vi "Traffic Monitoring Hub.vi"() -> ()   [LabVIEW 2017]
uses:
  <vilib>/LabVIEW Open Source Project/MQTT Broker/Client/Client.lvclass
  C:/Program Files (x86)/National Instruments/LabVIEW 2017/vi.lib/LabVIEW Open Source Project/MQTT Broker/MQTT_Base/MQTT_Base.lvclass
  <vilib>/LabVIEW Open Source Project/MQTT Broker/Control Packets/PUBLISH/PUBLISH.lvclass
  C:/Program Files (x86)/National Instruments/LabVIEW 2017/vi.lib/LabVIEW Open Source Project/MQTT Broker/Control Packets/ControlPacket/ControlPacket.lvclass
  <vilib>/LabVIEW Open Source Project/MQTT Broker/Client/Client.lvclass/Client.ctl
  <vilib>/LabVIEW Open Source Project/MQTT Broker/Control Packets/ControlPacket/ControlPacket.lvclass/ControlPacket.ctl
  0d705227-134d-4031-8d1e-e35da49b8ba8.vi
  89a43b97-b5cf-4dc9-9f30-016ac9be9430.vi
  45bbbbd6-bbd6-4c9d-8aa1-54a553140d59.vi
  b830538a-2e83-4cc7-9605-dce1a29f0d38.vi
  <vilib>/LabVIEW Open Source Project/MQTT Broker/MQTT_Base/Decode Publish Package.vi
  <vilib>/LabVIEW Open Source Project/MQTT Broker/MQTT_Base/MQTT_Base.lvclass
  <vilib>/LabVIEW Open Source Project/MQTT Broker/Control Packets/ControlPacket/ControlPacket.lvclass
panel:
  in  "Destroy Sim Cars":bool
  in  "Generate Sim Cars":bool
  in  "# Cars":i32=10
  out "Will Message":string
  out "last update":timestamp
  out "Payload":variant
  in  "State History":i32(listbox)
  out "Topic":string
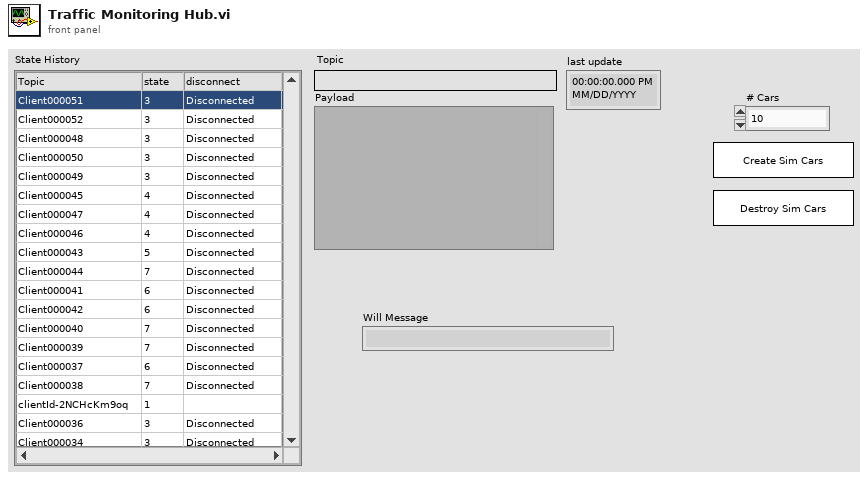
[diagram p1: front panel]
types:
  T1 = enum32{"Invalid", "Standard", "Closed", "Hidden", "Minimized", "Maximized"}
  T2 = enum32{"invalid app kind", "Development System", "Run Time System", "Student Edition", "Embedded LabVIEW", "Evaluation", "Custom"}
  T3 = cluster{"Core":cluster{"Current VI Reference":refnum<vi>, "Close Panel on Exit?":bool}, "server address":string, "project namespace":string, "Client Name":string, "Client":refnum<class "Client.lvclass">, "Close on MQTT Disconnection?":bool, "Subscription":string, "AppMessage":refnum<class "PUBLISH.lvclass">, "stop signal":refnum<user-event>}
  T4 = cluster{"Current VI Reference":refnum<vi>, "Close Panel on Exit?":bool}
  T5 = typedef "MQTT Server.lvlib/Client.lvclass/Public Events -- cluster.ctl" = cluster{"Connection Status":refnum<user-event>, "Connected":refnum<user-event>, "Application Message":refnum<user-event>}
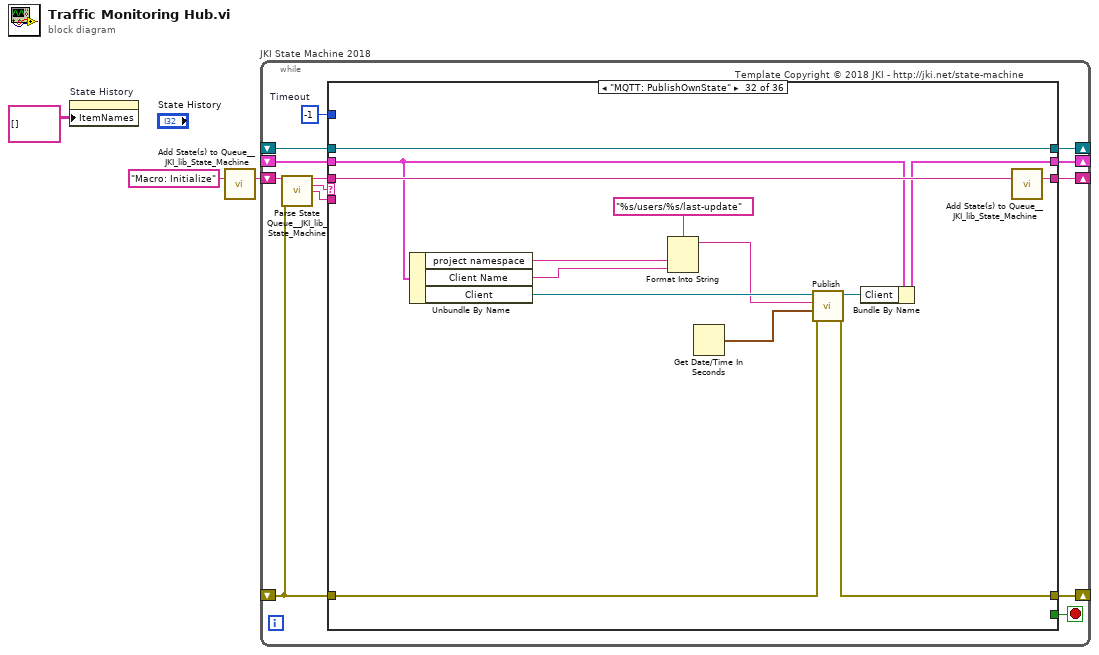
[diagram p0: block diagram]
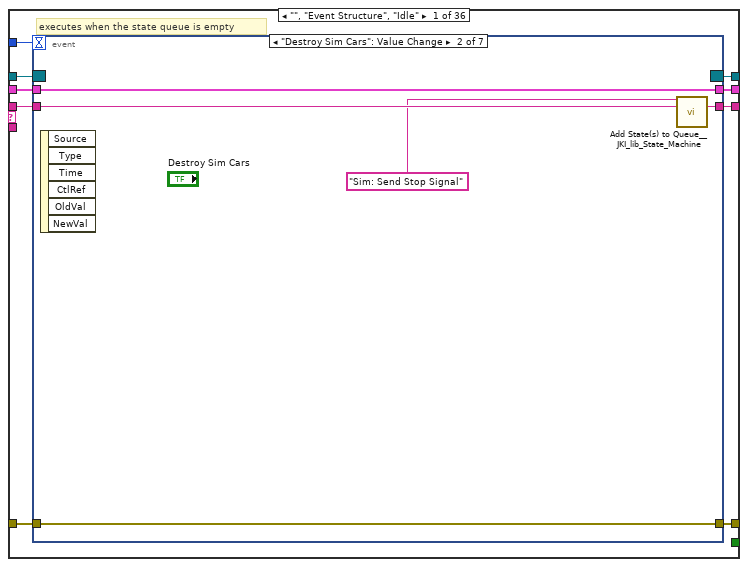
[diagram p2: hidden frame]
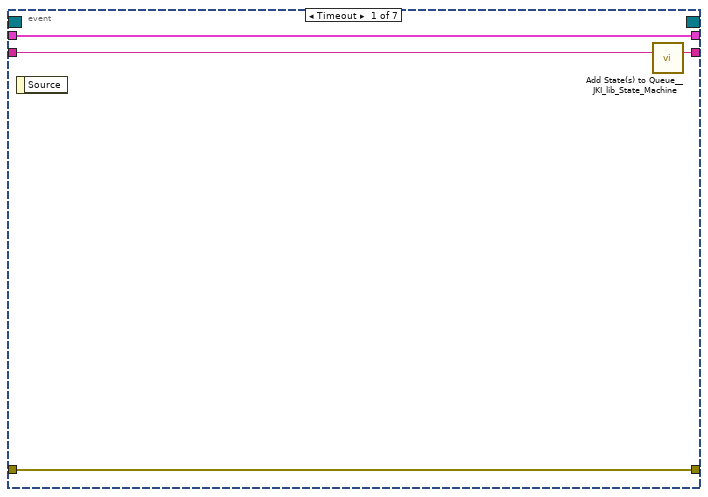
[diagram p3: hidden frame]
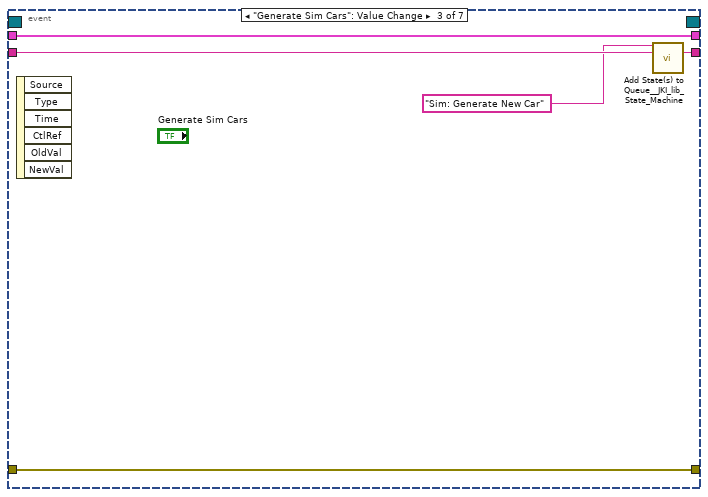
[diagram p4: hidden frame]
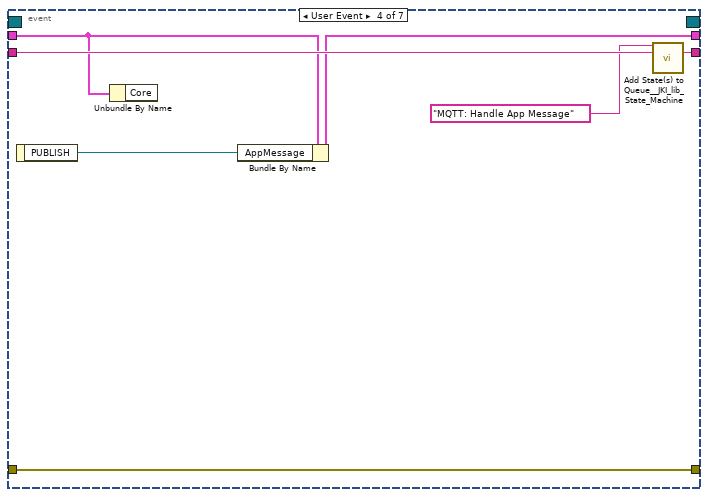
[diagram p5: hidden frame]
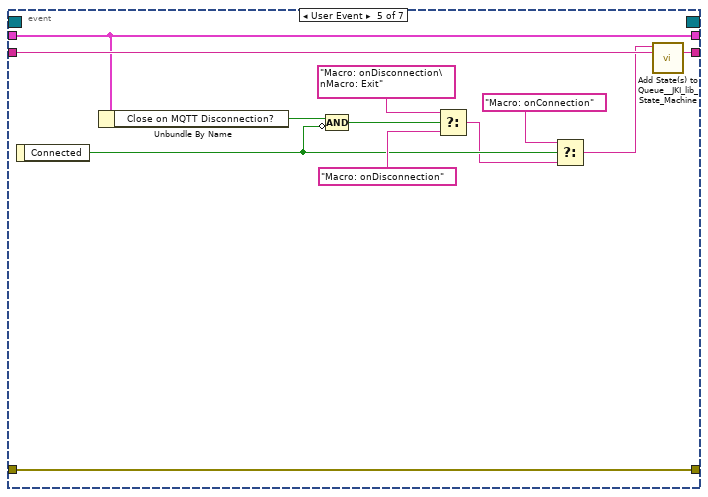
[diagram p6: hidden frame]
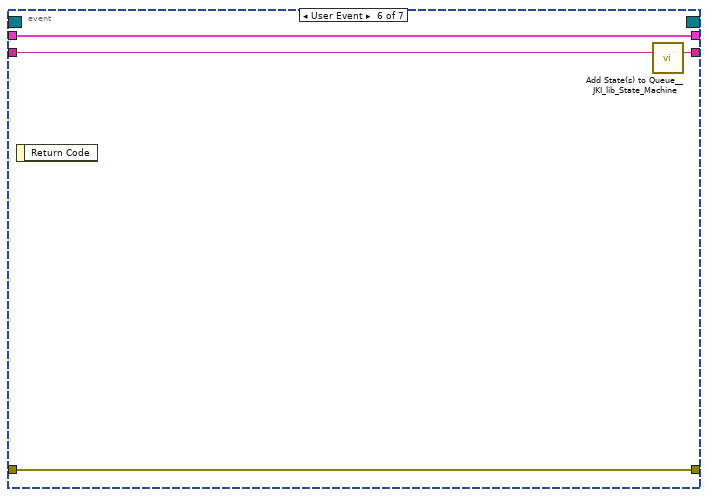
[diagram p7: hidden frame]
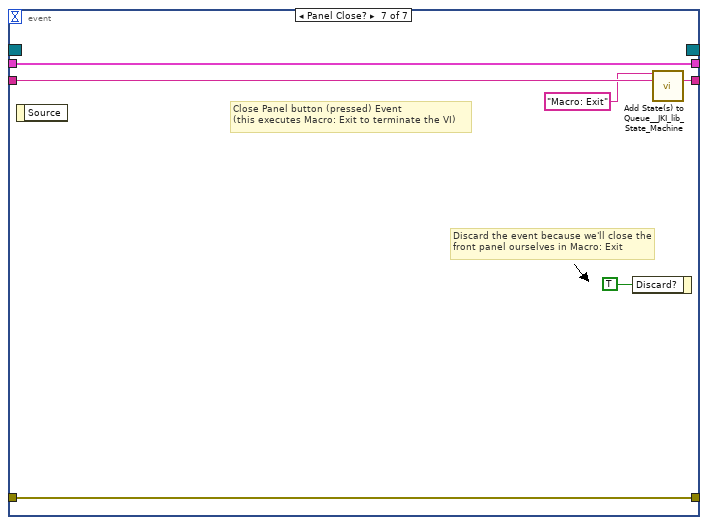
[diagram p8: hidden frame]
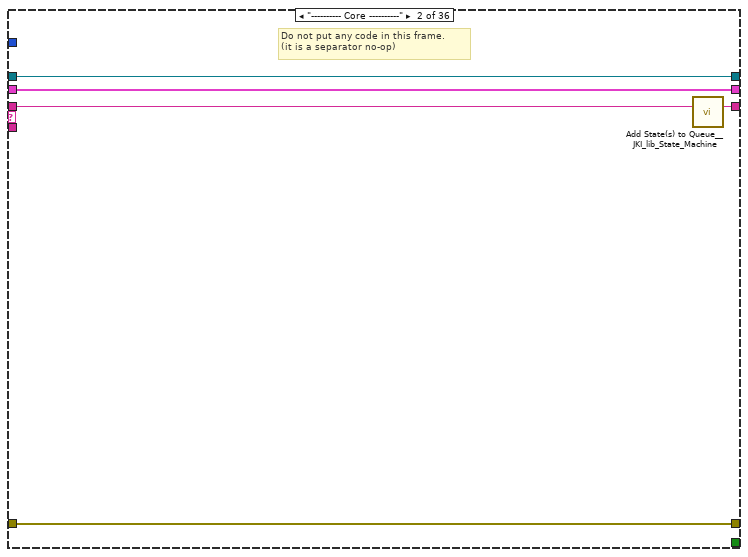
[diagram p9: hidden frame]
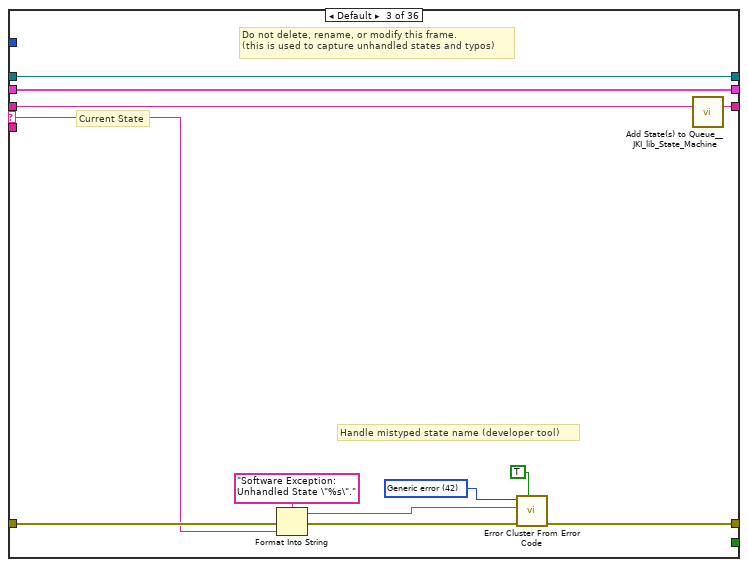
[diagram p10: hidden frame]
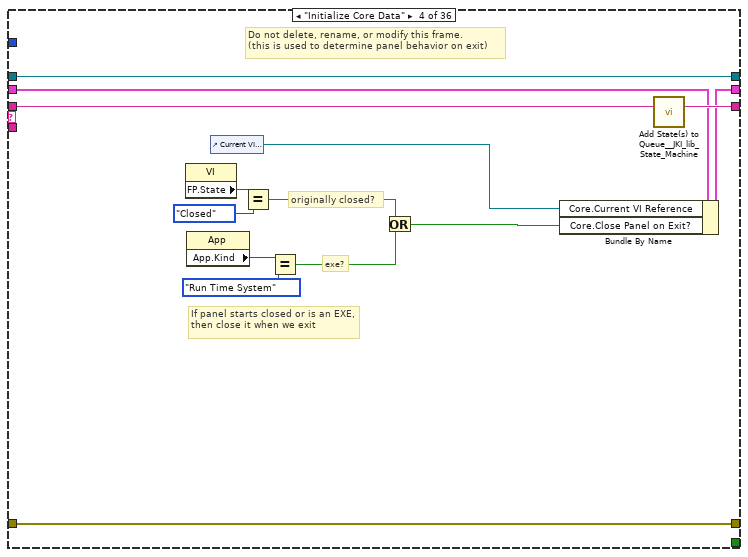
[diagram p11: hidden frame]
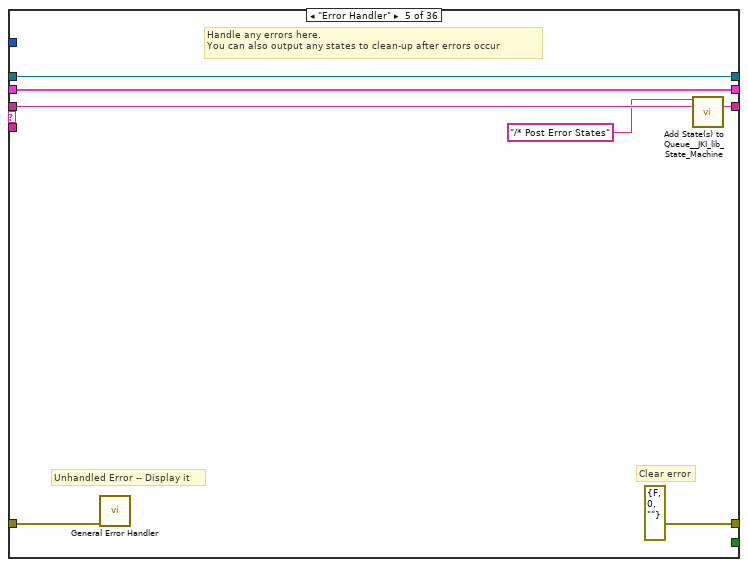
[diagram p12: hidden frame]
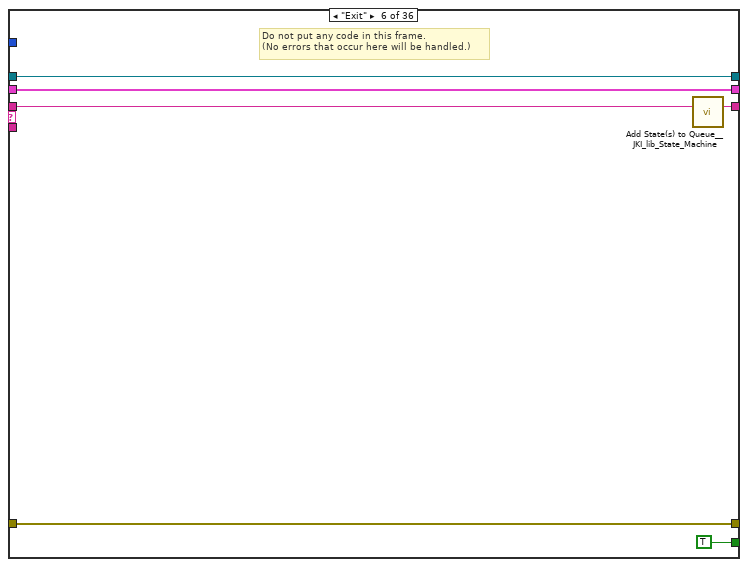
[diagram p13: hidden frame]
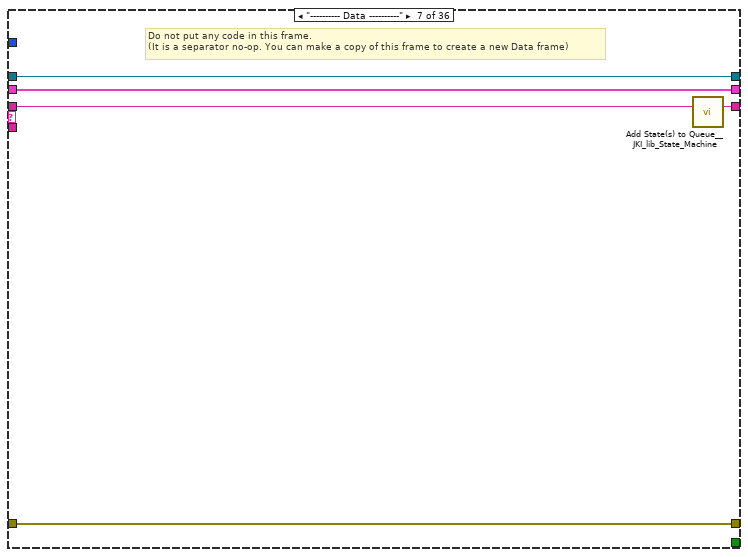
[diagram p14: hidden frame]
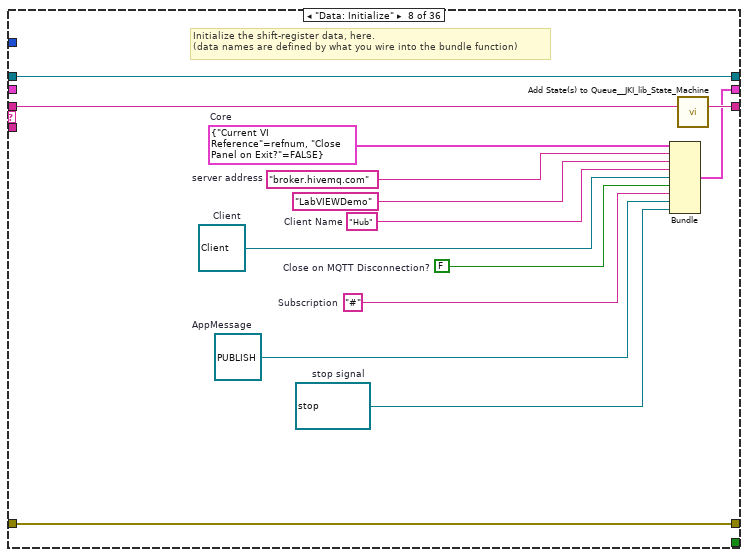
[diagram p15: hidden frame]
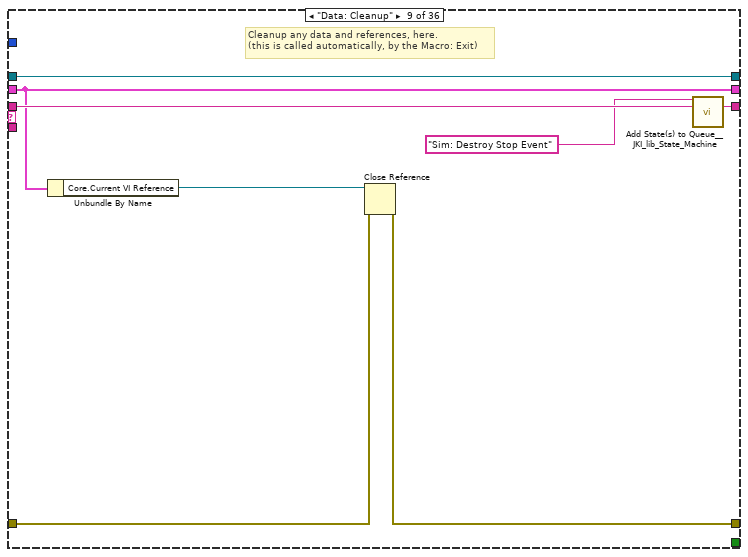
[diagram p16: hidden frame]
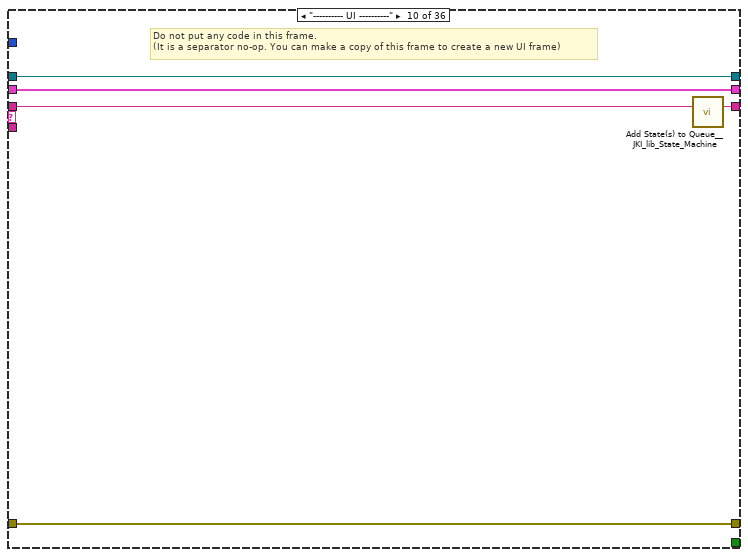
[diagram p17: hidden frame]
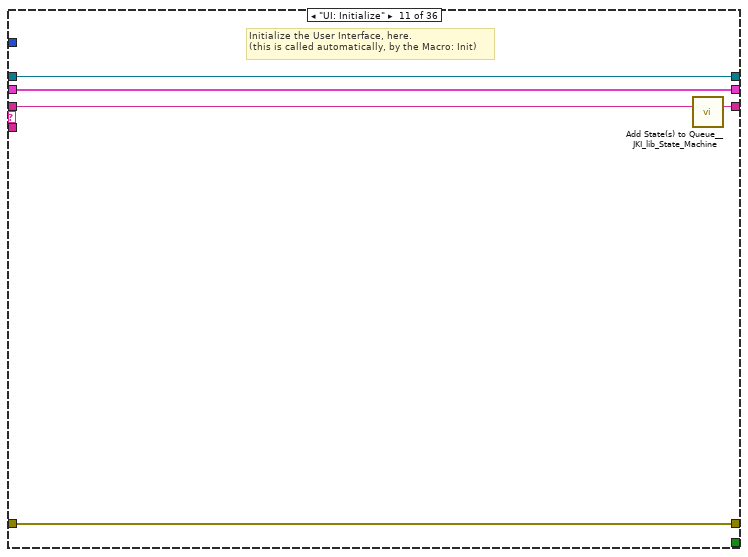
[diagram p18: hidden frame]
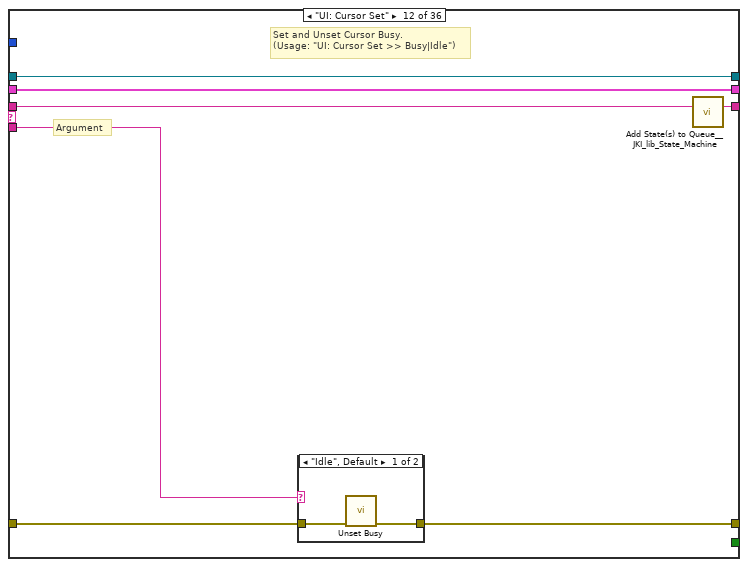
[diagram p19: hidden frame]
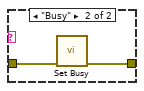
[diagram p20: hidden frame]
diagram:
  n1 = property on="State History" class="MCListbox (strict)"("ItemNames"=string[][] [] ("Item Names")) -> ()  [unwired: 2 in, 2 out]
  n2 = call <vilib>:"Add State(s) to Queue__JKI_lib_State_Machine.vi"("State(s) in (\"\")"="Macro: Initialize") -> ("States Out"=w2:string)  [unwired: 14 in]
  n3 = while "JKI State Machine 2018" {
    shift-right: [w9] -> _
    shift-left: _ -> [w8]
    shift-right: [w12] -> _
    shift-left: _ -> [w6]
    shift-right: [w11] -> _
    shift-left: w2 -> [w13]
    shift-right: [w4] -> _
    shift-left: _ -> [w5]
    stop <- w10 stop-if-true
    w7 = -1  # Timeout
    # "Template Copyright © 2018 JKI - http://jki.net/state-machine"
    n4 = call <vilib>:"Parse State Queue__JKI_lib_State_Machine.vi"("State Queue"=w13, "Error In (no error)"=w6) -> ("Remaining States"=w15:string, "Current State"=w16:string, "Arguments"=w14:string)  [unwired: 11 in]
    n5 = case shown="\"MQTT: PublishOwnState\"" w16 {
      selector: w16 -> [_ _ w75 _ _ _ _ _ _ _ _ _ _ _ _ _ _ _ _ _ _ _ _ _ _ _ _ _ _ _ _ _ _ _ _ _]
      tunnel: w15 -> [w25 w73 w79 w99 w106 w112 w117 w131 w139 w144 w149 w156 w168 w238 w244 w250 w256 w262 w268 w280 w285 w293 w299 w306 w317 w339 w347 w358 w370 w383 w396 w410 w424 w521 w527 w534]
      tunnel: w14 -> [_ _ _ _ _ _ _ _ _ _ _ w151 w162 _ _ _ _ _ _ _ _ _ _ _ _ _ _ _ _ _ _ _ _ _ _ _]
      tunnel: w8 -> [w23 w70 w77 w92 w103 w110 w114 _ w134 w141 w147 w154 w164 w235 w241 w247 w253 w259 w265 w277 w282 w287 w295 w302 w313 w336 w344 w355 w367 w380 w393 w407 w421 w518 w522 w532]
      tunnel: [w22 w71 w81 w96 errorcluster {"status"=FALSE, "code"=0, "source"=""} ("error out") w109 w115 w128 w135 w142 w146 w152 w165 w236 w242 w248 w254 w260 w266 w278 w283 w291 w297 w304 w315 w337 w341 w348 w360 w372 w388 w398 w420 w513 w523 w529] -> w12
      tunnel: w6 -> [w21 w71 w80 w96 w102 w109 w115 w128 w136 w142 w146 w153 w166 w236 w242 w248 w254 w260 w266 w278 w283 w291 w297 w304 w315 w337 w342 w351 w361 w373 w389 w399 w420 w511 w524 w530]
      tunnel: [w24 w72 w78 w98 w105 w111 w116 w130 w138 w143 w148 w155 w167 w237 w243 w249 w255 w261 w267 w279 w284 w292 w298 w305 w316 w338 w346 w357 w369 w382 w395 w409 w423 w520 w526 w533] -> w11
      tunnel: [_ _ _ _ _ TRUE _ _ _ _ _ _ _ _ _ _ _ _ _ _ _ _ _ _ _ _ _ _ _ _ _ _ _ _ _ _] -> w10
      tunnel: [w20 w70 w77 w97 w103 w110 w114 w129 w134 w141 w147 w154 w164 w235 w241 w247 w253 w259 w265 w277 w282 w286 w295 w302 w313 w336 w343 w356 w368 w381 w394 w408 w421 w519 w522 w532] -> w9
      tunnel: w7 -> [w19 _ _ _ _ _ _ _ _ _ _ _ _ _ _ _ _ _ _ _ _ _ _ _ _ _ _ _ _ _ _ _ _ _ _ _]
      tunnel: w5 -> [w18 w69 w74 w86 w100 w107 w113 w122 w133 w140 w145 w150 w161 w234 w239 w245 w251 w257 w263 w269 w281 w290 w296 w303 w314 w335 w340 _ w366 w379 w392 w406 w422 w517 w525 w528]
      tunnel: [w17 w69 w74 w86 w100 w107 w113 w122 w133 w140 w145 w150 w161 w234 w239 w245 w251 w257 w263 w269 w281 w290 w296 w303 w314 w335 w340 w350 w366 w379 w392 w406 w422 w517 w525 w528] -> w4
      frame "", "Event Structure", "Idle" {
        # "executes when the state queue is empty"
        n6 = event shown="[1] \"Destroy Sim Cars\": Value Change" {
          selector: w18 -> [_ _ _ _ _ _ _]
          dyn-events: [_ _ _ _ _ _ _] -> w17
          timeout: w19 -> [_ _ _ _ _ _ _]
          tunnel: w25 -> [w29 w34 w39 w46 w58 w62 w68]
          tunnel: [w28 w33 w38 w45 w57 w61 w67] -> w24
          tunnel: w23 -> [w26 w31 w36 w42 w55 w59 w65]
          tunnel: [w27 w32 w37 w44 w56 w60 w66] -> w22
          tunnel: w21 -> [w27 w32 w37 w44 w56 w60 w66]
          tunnel: [w26 w31 w36 w41 w55 w59 w65] -> w20
          event Timeout {
            n7 = event-data() -> ()  [unwired: 1 in, 1 out]
            n8 = call <vilib>:"Add State(s) to Queue__JKI_lib_State_Machine.vi"("State(s) in (\"\")"=w29) -> ("States Out"=w28:string)  [unwired: 14 in]
          }
          event "Destroy Sim Cars": Value Change {
            n9 = event-data() -> ()  [unwired: 1 in, 6 out]
            n10 = call <vilib>:"Add State(s) to Queue__JKI_lib_State_Machine.vi"("State(s) in Front (\"\")"="Sim: Send Stop Signal", "State(s) in (\"\")"=w34) -> ("States Out"=w33:string)  [unwired: 13 in]
          }
          event "Generate Sim Cars": Value Change {
            n11 = event-data() -> ()  [unwired: 1 in, 6 out]
            n12 = call <vilib>:"Add State(s) to Queue__JKI_lib_State_Machine.vi"("State(s) in Front (\"\")"="Sim: Generate New Car", "State(s) in (\"\")"=w39) -> ("States Out"=w38:string)  [unwired: 13 in]
          }
          event User Event {
            n13 = event-data() -> ("PUBLISH"=w43:refnum<class "PUBLISH.lvclass">)  [unwired: 1 in]
            n14 = Unbundle By Name(w42) -> ()  [unwired: 1 out]
            n15 = Bundle By Name(cluster=w42, "AppMessage"=w43) -> (w41:T3)
            n16 = call <vilib>:"Add State(s) to Queue__JKI_lib_State_Machine.vi"("State(s) in Front (\"\")"="MQTT: Handle App Message", "State(s) in (\"\")"=w46) -> ("States Out"=w45:string)  [unwired: 13 in]
          }
          event User Event {
            n17 = event-data() -> ("Connected"=w50:bool)  [unwired: 1 in]
            n18 = Unbundle By Name(w55) -> ("Close on MQTT Disconnection?"=w54:bool)
            n19 = Compound Arithmetic op=AND(w54, invert w50) -> (w53:bool)
            n20 = Select(t="Macro: onDisconnection\nMacro: Exit", s=w53, f="Macro: onDisconnection" ("t")) -> (s? t:f=w48:string)
            n21 = Select(t="Macro: onConnection", s=w50, f=w48) -> (s? t:f=w47:string)
            n22 = call <vilib>:"Add State(s) to Queue__JKI_lib_State_Machine.vi"("State(s) in Front (\"\")"=w47, "State(s) in (\"\")"=w58) -> ("States Out"=w57:string)  [unwired: 13 in]
          }
          event User Event {
            n23 = event-data() -> ()  [unwired: 1 in, 1 out]
            n24 = call <vilib>:"Add State(s) to Queue__JKI_lib_State_Machine.vi"("State(s) in (\"\")"=w62) -> ("States Out"=w61:string)  [unwired: 14 in]
          }
          event Panel Close? {
            # "Discard the event because we'll close the front panel ourselves in Macro: Exit"
            # "Close Panel button (pressed) Event\n(this executes Macro: Exit to terminate the VI)"
            n25 = event-data() -> ()  [unwired: 1 in, 1 out]
            n26 = event-data("Discard?"=TRUE) -> ()  [unwired: 1 in, 1 out]
            n27 = call <vilib>:"Add State(s) to Queue__JKI_lib_State_Machine.vi"("State(s) in Front (\"\")"="Macro: Exit", "State(s) in (\"\")"=w68) -> ("States Out"=w67:string)  [unwired: 13 in]
          }
        }
      }
      frame "---------- Core ----------" {
        # "Do not put any code in this frame.\n(it is a separator no-op)"
        n28 = call <vilib>:"Add State(s) to Queue__JKI_lib_State_Machine.vi"("State(s) in (\"\")"=w73) -> ("States Out"=w72:string)  [unwired: 14 in]
      }
      frame Default {
        w84 = 42 items=["No error", "Argument error", "Memory is full", "Out of zone", "End of file", "File already open", "Generic file I/O error", "File not found", "File permission error", "Disk is full", "Duplicate path", "Too many files open", "System feature not enabled", "Resource file not found", "Cannot add resource", "Resource not found", "Image not found", "Image memory error", "Pen does not exist", "Config type invalid", "Config token not found", "Config parse error", "Config memory error", "Bad external code format", "Bad external code offset", "External code not present", "Null window", "Destroy window error", "Null menu", "Print aborted", "Bad print record", "Print driver error", "Windows error during printing", "Memory error during printing", "Print dialog error", "Generic print error", "Invalid device refnum", "Device not found", "Device parameter error", "Device unit error", "Cannot open device", "Device call aborted", "Generic error", "Cancelled by user", "Object ID too low", "Object ID too high", "Object not in heap", "Unknown heap", "Unknown object (invalid DefProc)", "Unknown object (DefProc not in table)", "Message out of range", "Invalid (null) method", "Unknown message", "Manager call not supported", "Bad address", "Network operation in progress", "Network operation timed out", "Connection is busy", "Network attribute not supported", "Network error", "Address in use", "System out of memory", "Connection aborted", "Connection refused", "Not connected", "Already connected", "Connection closed", "Initialization error (interapplication manager)", "Bad occurrence", "Wait on unbound occurrence handler", "Occurrence queue overflow", "Datalog type conflict", "Unused", "Unrecognized type (interapplication manager)", "Memory corrupt", "Failed to make temporary DLL", "Old CIN version", "Drag socket not found", "Failed to load drop-object", "Failed to register OLE object", "Failed to release OLE object", "Format specifier type mismatch", "Unknown format specifier", "Too few format specifiers", "Too many format specifiers", "Scan failed", "Newer CIN version", "Error converting to variant", "Runtime menu error", "Password tampered", "Variant attribute not found", "Incompatible variant data type", "Event data is not available", "Event Store is not present", "Occurrence is not found", "Event Queue is not created", "Event info is not available", "Refnum passed is NULL", "Error retrieving Class GUID", "Error retrieving CoClass GUID", "Error retrieving TypeLib GUID.", "Bad built application magic bytes.", "Specific driver is different from the specific driver associated with the Logical Name.", "There is no session opened to the class driver.", "Max Error", "MAX - Error with config objects", "MAX - Error loading configuration", "MAX - Group not supported"]
        # "Current State"
        # "Do not delete, rename, or modify this frame.\n(this is used to capture unhandled states and typos)"
        # "Handle mistyped state name (developer tool)"
        n29 = Format Into String(format string="Software Exception: Unhandled State \"%s\"." ("message"), error in=w80, w75) -> (resulting string=w83:string, error out=w82:errorcluster)  [unwired: 1 in]
        n30 = call <vilib>:"Error Cluster From Error Code.vi"("show call chain? (False)"=TRUE, "error in (no error)"=w82, "error message (\"\")"=w83, "error code (0)"=w84) -> ("error out"=w81:errorcluster)  [unwired: 5 in]
        n31 = call <vilib>:"Add State(s) to Queue__JKI_lib_State_Machine.vi"("State(s) in (\"\")"=w79) -> ("States Out"=w78:string)  [unwired: 14 in]
      }
      frame "Initialize Core Data" {
        # "Do not delete, rename, or modify this frame.\n(this is used to determine panel behavior on exit)"
        # "originally closed?"
        # "exe?"
        # "If panel starts closed or is an EXE, then close it when we exit"
        n32 = property class="VI"() -> ("FP.State"=w89:T1)  [unwired: 2 in, 2 out]
        n33 = property class="App"() -> ("App.Kind"=w95:T2)  [unwired: 2 in, 2 out]
        n34 = control-ref of="Current VI Reference"() -> (w90:refnum<vi>)
        n35 = Equal?(x=w89, y=T1."Closed" ("Front Panel Window:State")) -> (x = y?=w87:bool)
        n36 = Equal?(x=w95, y=T2."Run Time System" ("Application:Kind")) -> (x = y?=w93:bool)
        n37 = Or(x=w87, y=w93) -> (x .or. y?=w91:bool)
        n38 = Bundle By Name(cluster=w92, "Core.Current VI Reference"=w90, "Core.Close Panel on Exit?"=w91) -> (w97:T3)
        n39 = call <vilib>:"Add State(s) to Queue__JKI_lib_State_Machine.vi"("State(s) in (\"\")"=w99) -> ("States Out"=w98:string)  [unwired: 14 in]
      }
      frame "Error Handler" {
        # "Unhandled Error -- Display it"
        # "Handle any errors here.\nYou can also output any states to clean-up after errors occur"
        # "Clear error"
        n40 = call <vilib>:"General Error Handler.vi"("error in (no error)"=w102) -> ()  [unwired: 10 in, 5 out]
        n41 = call <vilib>:"Add State(s) to Queue__JKI_lib_State_Machine.vi"("State(s) in Front (\"\")"="/* Post Error States", "State(s) in (\"\")"=w106) -> ("States Out"=w105:string)  [unwired: 13 in]
      }
      frame "Exit" {
        # "Do not put any code in this frame.\n(No errors that occur here will be handled.)"
        n42 = call <vilib>:"Add State(s) to Queue__JKI_lib_State_Machine.vi"("State(s) in (\"\")"=w112) -> ("States Out"=w111:string)  [unwired: 14 in]
      }
      frame "---------- Data ----------" {
        # "Do not put any code in this frame.\n(It is a separator no-op. You can make a copy of this frame to create a new Data frame)"
        n43 = call <vilib>:"Add State(s) to Queue__JKI_lib_State_Machine.vi"("State(s) in (\"\")"=w117) -> ("States Out"=w116:string)  [unwired: 14 in]
      }
      frame "Data: Initialize" {
        w118 = refnum<user-event> refnum  # stop signal
        w119 = refnum<class "PUBLISH.lvclass"> refnum  # AppMessage
        w120 = "#"  # Subscription
        w121 = FALSE  # Close on MQTT Disconnection?
        w123 = refnum<class "Client.lvclass"> refnum  # Client
        w124 = "broker.hivemq.com"  # server address
        w126 = T4 {"Current VI Reference"=refnum, "Close Panel on Exit?"=FALSE}  # Core
        w127 = "Hub"  # Client Name
        # "Initialize the shift-register data, here.\n(data names are defined by what you wire into the bundle function)"
        n44 = Bundle("Core"=w126, "server address"=w124, "project namespace"="LabVIEWDemo", "Client Name"=w127, "Client"=w123, "Close on MQTT Disconnection?"=w121, "Subscription"=w120, "AppMessage"=w119, "stop signal"=w118) -> (w129:T3)  [unwired: 1 in]
        n45 = call <vilib>:"Add State(s) to Queue__JKI_lib_State_Machine.vi"("State(s) in (\"\")"=w131) -> ("States Out"=w130:string)  [unwired: 14 in]
      }
      frame "Data: Cleanup" {
        # "Cleanup any data and references, here.\n(this is called automatically, by the Macro: Exit)"
        n46 = Unbundle By Name(w134) -> ("Core.Current VI Reference"=w137:refnum<vi>)
        n47 = Close Reference(reference=w137, error in (no error)=w136) -> (error out=w135:errorcluster)
        n48 = call <vilib>:"Add State(s) to Queue__JKI_lib_State_Machine.vi"("State(s) in Front (\"\")"="Sim: Destroy Stop Event", "State(s) in (\"\")"=w139) -> ("States Out"=w138:string)  [unwired: 13 in]
      }
      frame "---------- UI ----------" {
        # "Do not put any code in this frame.\n(It is a separator no-op. You can make a copy of this frame to create a new UI frame)"
        n49 = call <vilib>:"Add State(s) to Queue__JKI_lib_State_Machine.vi"("State(s) in (\"\")"=w144) -> ("States Out"=w143:string)  [unwired: 14 in]
      }
      frame "UI: Initialize" {
        # "Initialize the User Interface, here.\n(this is called automatically, by the Macro: Init)"
        n50 = call <vilib>:"Add State(s) to Queue__JKI_lib_State_Machine.vi"("State(s) in (\"\")"=w149) -> ("States Out"=w148:string)  [unwired: 14 in]
      }
      frame "UI: Cursor Set" {
        # "Argument"
        # "Set and Unset Cursor Busy.\n(Usage: \"UI: Cursor Set >> Busy|Idle\")"
        n51 = case shown="\"Idle\", Default" w151 {
          tunnel: w153 -> [w158 w160]
          tunnel: [w157 w159] -> w152
          frame "Idle", Default {
            n52 = call <vilib>:"Unset Busy.vi"("error in (no error)"=w158) -> ("error out"=w157:errorcluster)  [unwired: 10 in]
          }
          frame "Busy" {
            n53 = call <vilib>:"Set Busy.vi"("error in (no error)"=w160) -> ("error out"=w159:errorcluster)  [unwired: 9 in, 1 out]
          }
        }
        n54 = call <vilib>:"Add State(s) to Queue__JKI_lib_State_Machine.vi"("State(s) in (\"\")"=w156) -> ("States Out"=w155:string)  [unwired: 14 in]
      }
      frame "UI: Front Panel State" {
        # "Argument"
        # "Set Front Panel Open or Closed\n(Usage: \"UI: Front Panel State >> Open|Close\")"
        n55 = Unbundle By Name(w164) -> ("Core.Current VI Reference"=w163:refnum<vi>)
        n56 = case shown="\"Minimize\", \"Minimized\"" w162 {
          tunnel: w166 -> [w174 w189 w200 w213 w226]
          tunnel: [w176 w190 w202 w215 w228] -> w165
          tunnel: w163 -> [w175 w187 w201 w214 w227]
          frame "Open", "Standard", Default {
            w169 = T1."Standard" ("State")
            n57 = property class="VI"(reference=w175, error in=w174) -> (reference out=w172:refnum<vi>, error out=w173:errorcluster, "FP.State"=w171:T1)
            n58 = Not Equal?(x=w171, y=w169) -> (x != y?=w170:bool)
            n59 = case shown="True" w170 {
              tunnel: [w180 w182] -> w176
              tunnel: w173 -> [w179 w182]
              tunnel: w172 -> [w178 _]
              tunnel: w169 -> [w177 _]
              frame True {
                n60 = invoke class="VI" method="FP.Open"(reference=w178, error in=w179, "Activate"=TRUE, "State"=w177) -> (error out=w180:errorcluster)  [unwired: 1 in, 4 out]
              }
              frame False {
              }
            }
          }
          frame "Close", "Closed" {
            n61 = property class="VI"(reference=w187, error in=w189) -> (reference out=w186:refnum<vi>, error out=w188:errorcluster, "FP.State"=w184:T1)
            n62 = Not Equal?(x=w184, y=T1."Closed" ("Front Panel Window:State")) -> (x != y?=w183:bool)
            n63 = case shown="True" w183 {
              tunnel: [w191 w194] -> w190
              tunnel: w188 -> [w191 w193]
              tunnel: w186 -> [_ w192]
              frame False {
              }
              frame True {
                n64 = invoke class="VI" method="FP.Close"(reference=w192, error in=w193) -> (error out=w194:errorcluster)  [unwired: 1 in, 2 out]
              }
            }
          }
          frame "Hidden", "Hide" {
            w195 = T1."Hidden" ("State")
            n65 = property class="VI"(reference=w201, error in=w200) -> (reference out=w198:refnum<vi>, error out=w199:errorcluster, "FP.State"=w197:T1)
            n66 = Not Equal?(x=w197, y=w195) -> (x != y?=w196:bool)
            n67 = case shown="True" w196 {
              tunnel: [w206 w207] -> w202
              tunnel: w199 -> [w205 w207]
              tunnel: w198 -> [w204 _]
              tunnel: w195 -> [w203 _]
              frame True {
                n68 = invoke class="VI" method="FP.Open"(reference=w204, error in=w205, "State"=w203) -> (error out=w206:errorcluster)  [unwired: 2 in, 4 out]
              }
              frame False {
              }
            }
          }
          frame "Minimize", "Minimized" {
            w208 = T1."Minimized" ("State")
            n69 = property class="VI"(reference=w214, error in=w213) -> (reference out=w211:refnum<vi>, error out=w212:errorcluster, "FP.State"=w210:T1)
            n70 = Not Equal?(x=w210, y=w208) -> (x != y?=w209:bool)
            n71 = case shown="True" w209 {
              tunnel: [w219 w220] -> w215
              tunnel: w212 -> [w218 w220]
              tunnel: w211 -> [w217 _]
              tunnel: w208 -> [w216 _]
              frame True {
                n72 = invoke class="VI" method="FP.Open"(reference=w217, error in=w218, "State"=w216) -> (error out=w219:errorcluster)  [unwired: 2 in, 4 out]
              }
              frame False {
              }
            }
          }
          frame "Maximize", "Maximized" {
            w221 = T1."Maximized" ("State")
            n73 = property class="VI"(reference=w227, error in=w226) -> (reference out=w224:refnum<vi>, error out=w225:errorcluster, "FP.State"=w223:T1)
            n74 = Not Equal?(x=w223, y=w221) -> (x != y?=w222:bool)
            n75 = case shown="True" w222 {
              tunnel: [w232 w233] -> w228
              tunnel: w225 -> [w231 w233]
              tunnel: w224 -> [w230 _]
              tunnel: w221 -> [w229 _]
              frame True {
                n76 = invoke class="VI" method="FP.Open"(reference=w230, error in=w231, "State"=w229) -> (error out=w232:errorcluster)  [unwired: 2 in, 4 out]
              }
              frame False {
              }
            }
          }
        }
        n77 = call <vilib>:"Add State(s) to Queue__JKI_lib_State_Machine.vi"("State(s) in (\"\")"=w168) -> ("States Out"=w167:string)  [unwired: 14 in]
      }
      frame "---------- Macro ----------" {
        # "Do not put any code in this frame.\n(It is a separator no-op. You can make a copy of this frame to create a new Macro frame)"
        n78 = call <vilib>:"Add State(s) to Queue__JKI_lib_State_Machine.vi"("State(s) in (\"\")"=w238) -> ("States Out"=w237:string)  [unwired: 14 in]
      }
      frame "Macro: Initialize" {
        w240 = "Data: Initialize\nInitialize Core Data\nUI: Initialize\nUI: Front Panel State >> Open\nSim: Create Stop Event\nMacro: MQTTConnect"  # Data: Initialize Initialize Core Data UI: Initialize UI: Front Panel State >> Open Sim: Create Stop Event Macro: MQTTConnect
        # "Initialization Macro\n(This is called once, when the VI starts)"
        n79 = call <vilib>:"Add State(s) to Queue__JKI_lib_State_Machine.vi"("State(s) in Front (\"\")"=w240, "State(s) in (\"\")"=w244) -> ("States Out"=w243:string)  [unwired: 13 in]
      }
      frame "Macro: MQTTConnect" {
        n80 = call <vilib>:"Add State(s) to Queue__JKI_lib_State_Machine.vi"("State(s) in Front (\"\")"="MQTT: Create Client\nMQTT: Register for Events\nMQTT: Connect", "State(s) in (\"\")"=w250) -> ("States Out"=w249:string)  [unwired: 13 in]
      }
      frame "Macro: onConnection" {
        n81 = call <vilib>:"Add State(s) to Queue__JKI_lib_State_Machine.vi"("State(s) in Front (\"\")"="MQTT: Subscribe\nMQTT: PublishOwnState", "State(s) in (\"\")"=w256) -> ("States Out"=w255:string)  [unwired: 13 in]
      }
      frame "Macro: onDisconnection" {
        n82 = call <vilib>:"Add State(s) to Queue__JKI_lib_State_Machine.vi"("State(s) in Front (\"\")"="", "State(s) in (\"\")"=w262) -> ("States Out"=w261:string)  [unwired: 13 in]
      }
      frame "Macro: MQTTDisconnect" {
        n83 = call <vilib>:"Add State(s) to Queue__JKI_lib_State_Machine.vi"("State(s) in Front (\"\")"="MQTT: Unsubscribe\nMQTT: Unregister\nMQTT: Disconnect\nMQTT: Destroy Client", "State(s) in (\"\")"=w268) -> ("States Out"=w267:string)  [unwired: 13 in]
      }
      frame "Macro: Exit" {
        # "Exit Macro\n(This is called once, when the VI exits)"
        n84 = Unbundle By Name(w277) -> ("Core.Close Panel on Exit?"=w276:bool)
        n85 = Select(t="UI: Front Panel State >> Close", s=w276, f="") -> (s? t:f=w273:string)
        n86 = call <vilib>:"Add State(s) to Queue__JKI_lib_State_Machine.vi"("State(s) in Front (\"\")"="Sim: Send Stop Signal\nMacro: MQTTDisconnect", "State(s) in (\"\")"=w273, "State(s) at Back (\"\")"="Data: Cleanup\nExit") -> ("States Out"=w271:string)  [unwired: 12 in]
        n87 = call <vilib>:"Add State(s) to Queue__JKI_lib_State_Machine.vi"("State(s) in Front (\"\")"=w271, "State(s) in (\"\")"=w280) -> ("States Out"=w279:string)  [unwired: 13 in]
      }
      frame "---------- Simulation ----------" {
        # "Simulation Separator\n(You can make a copy of, or modify, this frame)"
        n88 = call <vilib>:"Add State(s) to Queue__JKI_lib_State_Machine.vi"("State(s) in (\"\")"=w285) -> ("States Out"=w284:string)  [unwired: 14 in]
      }
      frame "Sim: Create Stop Event" {
        w289 = FALSE  # stop
        n89 = Create User Event(user event datatype=w289) -> (user event=w288:refnum<user-event>)  [unwired: 1 in, 1 out]
        n90 = Bundle By Name(cluster=w287, "stop signal"=w288) -> (w286:T3)
        n91 = call <vilib>:"Add State(s) to Queue__JKI_lib_State_Machine.vi"("State(s) in (\"\")"=w293) -> ("States Out"=w292:string)  [unwired: 14 in]
      }
      frame "Sim: Destroy Stop Event" {
        n92 = Unbundle By Name(w295) -> ("stop signal"=w294:refnum<user-event>)
        n93 = Destroy User Event(user event=w294) -> ()  [unwired: 1 in, 1 out]
        n94 = call <vilib>:"Add State(s) to Queue__JKI_lib_State_Machine.vi"("State(s) in (\"\")"=w299) -> ("States Out"=w298:string)  [unwired: 14 in]
      }
      frame "Sim: Send Stop Signal" {
        n95 = Unbundle By Name(w302) -> ("stop signal"=w301:refnum<user-event>)
        n96 = Generate User Event(user event=w301, event data cluster=TRUE ("event data")) -> ()  [unwired: 2 in, 2 out]
        n97 = call <vilib>:"Add State(s) to Queue__JKI_lib_State_Machine.vi"("State(s) in (\"\")"=w306) -> ("States Out"=w305:string)  [unwired: 14 in]
      }
      frame "Sim: Generate New Car" {
        n98 = Unbundle By Name(w313) -> ("stop signal"=w308:refnum<user-event>, "project namespace"=w307:string)
        n99 = vi-ref "Simulated Client.vi"() -> (w310:refnum<vi>)
        n100 = property class="VI Interface Type 6"(reference=w310) -> (reference out=w312:refnum<vi>, "Name"=w311:string)  [unwired: 1 in, 1 out]
        n101 = for {
          N: "# Cars" -> [_]
          tunnel: w311 -> [w333]
          tunnel: w312 -> [w331]
          tunnel: w308 -> [w330]
          shift-right: [w320] -> _
          shift-left: _ -> [w322]
          tunnel: w307 -> [w319]
          n102 = Open VI Reference(type specifier VI Refnum (for type only)=w331, vi path=w333, options=192) -> (vi reference=w332:refnum<vi>)  [unwired: 3 in, 1 out]
          n103 = Format Into String(format string="Client%06d", w322) -> (resulting string=w329:string)  [unwired: 2 in, 1 out]
          n104 = Random Number (0-1)() -> (number: 0 to 1=w327:dbl)
          n105 = Multiply(x=500.0, y=w327) -> (x*y=w325:dbl)
          n106 = Add(x=w325, y=1000 ("period (ms)")) -> (x+y=w323:dbl)
          n107 = To Long Integer(number=w323) -> (32bit integer=w318:i32)
          n108 = call-by-ref "Start Asynchronous Call"(reference=w332, "Stop Signal"=w330, "period (ms)"=w318, "Client Name"=w329, "project namespace"=w319) -> ()  [unwired: 9 in, 2 out]
          n109 = Increment(x=w322) -> (x+1=w321:u32)
          n110 = To Unsigned Long Integer(number=w321) -> (unsigned 32bit integer=w320:u32)
        }
        n111 = call <vilib>:"Add State(s) to Queue__JKI_lib_State_Machine.vi"("State(s) in (\"\")"=w317) -> ("States Out"=w316:string)  [unwired: 14 in]
      }
      frame "---------- MQTT ----------" {
        # "MQTT Separator\n(You can make a copy of, or modify, this frame)"
        n112 = call <vilib>:"Add State(s) to Queue__JKI_lib_State_Machine.vi"("State(s) in (\"\")"=w339) -> ("States Out"=w338:string)  [unwired: 14 in]
      }
      frame "MQTT: Create Client" {
        n113 = call <vilib>:"Create MQTT Client.vi"("error in (no error)"=w342) -> ("error out"=w341:errorcluster, "Client out"=w345:refnum<class "Client.lvclass">)  [unwired: 9 in]
        n114 = Bundle By Name(cluster=w344, "Client"=w345) -> (w343:T3)
        n115 = call <vilib>:"Add State(s) to Queue__JKI_lib_State_Machine.vi"("State(s) in (\"\")"=w347) -> ("States Out"=w346:string)  [unwired: 14 in]
      }
      frame "MQTT: Register for Events" {
        n116 = Unbundle By Name(w355) -> ("Client"=w353:refnum<class "Client.lvclass">)
        n117 = call <vilib>:"Read Public Events.vi"("error in (no error)"=w351, "Client in"=w353) -> ("error out"=w349:errorcluster, "Client Public Events"=w354:T5, "Client out"=w352:refnum<class "Client.lvclass">)  [unwired: 7 in]
        n118 = register-events(error in=w349, w354) -> (reference out=w350:refnum<event-registration>, error out=w348:errorcluster)  [unwired: 1 in]
        n119 = Bundle By Name(cluster=w355, "Client"=w352) -> (w356:T3)
        n120 = call <vilib>:"Add State(s) to Queue__JKI_lib_State_Machine.vi"("State(s) in (\"\")"=w358) -> ("States Out"=w357:string)  [unwired: 14 in]
      }
      frame "MQTT: Connect" {
        n121 = Unbundle By Name(w367) -> ("server address"=w359:string, "Client"=w363:refnum<class "Client.lvclass">)
        n122 = call <vilib>:"Start.vi"("error in (no error)"=w361, "MQTT_Base in"=w363) -> ("error out"=w365:errorcluster, "MQTT_Base out"=w364:refnum<class "Client.lvclass">)  [unwired: 7 in, 1 out]
        n123 = call <vilib>:"Connect to Server.vi"("error in (no error)"=w365, "address (localhost)"=w359, "Client in"=w364) -> ("error out"=w360:errorcluster, "Client out"=w362:refnum<class "Client.lvclass">)  [unwired: 5 in, 2 out]
        n124 = Bundle By Name(cluster=w367, "Client"=w362) -> (w368:T3)
        n125 = call <vilib>:"Add State(s) to Queue__JKI_lib_State_Machine.vi"("State(s) in (\"\")"=w370) -> ("States Out"=w369:string)  [unwired: 14 in]
      }
      frame "MQTT: Subscribe" {
        n126 = Unbundle By Name(w380) -> ("project namespace"=w377:string, "Subscription"=w376:string, "Client"=w375:refnum<class "Client.lvclass">)
        n127 = Format Into String(format string="%s/%s", w377, w376) -> (resulting string=w371:string)  [unwired: 2 in, 1 out]
        n128 = call <vilib>:"Subscribe (SingleTopic).vi"("error in (no error)"=w373, "Topic Filter"=w371, "MQTT_Base in"=w375) -> ("error out"=w372:errorcluster, "MQTT_Base out"=w374:refnum<class "Client.lvclass">)  [unwired: 7 in]
        n129 = Bundle By Name(cluster=w380, "Client"=w374) -> (w381:T3)
        n130 = call <vilib>:"Add State(s) to Queue__JKI_lib_State_Machine.vi"("State(s) in (\"\")"=w383) -> ("States Out"=w382:string)  [unwired: 14 in]
      }
      frame "MQTT: Unsubscribe" {
        n131 = Unbundle By Name(w393) -> ("project namespace"=w386:string, "Subscription"=w384:string, "Client"=w391:refnum<class "Client.lvclass">)
        n132 = Format Into String(format string="%s/%s", w386, w384) -> (resulting string=w385:string)  [unwired: 2 in, 1 out]
        n133 = call <vilib>:"Unsubscribe (SingleTopic).vi"("error in (no error)"=w389, "Topic Filter"=w385, "MQTT_Base in"=w391) -> ("error out"=w388:errorcluster, "MQTT_Base out"=w390:refnum<class "Client.lvclass">)  [unwired: 7 in]
        n134 = Bundle By Name(cluster=w393, "Client"=w390) -> (w394:T3)
        n135 = call <vilib>:"Add State(s) to Queue__JKI_lib_State_Machine.vi"("State(s) in (\"\")"=w396) -> ("States Out"=w395:string)  [unwired: 14 in]
      }
      frame "MQTT: PublishOwnState" {
        n136 = Unbundle By Name(w407) -> ("project namespace"=w402:string, "Client Name"=w401:string, "Client"=w404:refnum<class "Client.lvclass">)
        n137 = Format Into String(format string="%s/users/%s/last-update", w402, w401) -> (resulting string=w400:string)  [unwired: 2 in, 1 out]
        n138 = Get Date/Time In Seconds() -> (seconds since 1Jan1904=w397:timestamp)
        n139 = call <vilib>:"Publish.vi"("error in (no error)"=w399, "Payload"=w397, "Topic Name (empty: Payload name)"=w400, "Client in"=w404) -> ("error out"=w398:errorcluster, "Client out"=w405:refnum<class "Client.lvclass">)  [unwired: 5 in, 1 out]
        n140 = Bundle By Name(cluster=w407, "Client"=w405) -> (w408:T3)
        n141 = call <vilib>:"Add State(s) to Queue__JKI_lib_State_Machine.vi"("State(s) in (\"\")"=w410) -> ("States Out"=w409:string)  [unwired: 14 in]
      }
      frame "MQTT: Handle App Message" {
        n142 = Unbundle By Name(w421) -> ("Client"=w415:refnum<class "Client.lvclass">, "AppMessage"=w417:refnum<class "PUBLISH.lvclass">)  [unwired: 1 out]
        n143 = call <vilib>:"getTopicName.vi"("PUBLISH in"=w417) -> ("Topic"=w414:string, "PUBLISH out"=w416:refnum<class "PUBLISH.lvclass">)  [unwired: 8 in, 1 out]
        "Topic" <- w414
        n144 = property on="State History" class="MCListbox (strict)"() -> ("ItemNames"=w412:string[][])  [unwired: 2 in, 2 out]
        n145 = call "topic_to_Array.vi"("Topic"=w414) -> ("Topic (Array)"=w419:string[])  [unwired: 10 in]
        n146 = Delete From Array(array=w419) -> (deleted portion=w418:string, array with subset deleted=w413:string[])  [unwired: 2 in]
        n147 = case shown="\"disconnect\"" w418 {
          tunnel: w416 -> [w427 w433 w446 w472 w487]
          tunnel: w415 -> [w428 w432 w445 w471 _]
          tunnel: w413 -> [_ _ w444 w470 w497]
          tunnel: w412 -> [w425 w429 w437 w463 w490]
          tunnel: [w425 w429 w436 w462 w489] -> w411
          frame Default {
            n148 = call "Decode Publish Packet.vim"("PUBLISH"=w427, "Client in"=w428) -> ("Payload"=→"Payload":variant)  [unwired: 6 in, 3 out]
          }
          frame "last-update" {
            n149 = Get Date/Time In Seconds() -> (seconds since 1Jan1904=w431:timestamp)
            n150 = call "Decode Publish Packet.vim"("Payload type"=w431, "PUBLISH"=w433, "Client in"=w432) -> ("Payload"=→"last update":timestamp)  [unwired: 5 in, 3 out]
          }
          frame "state" {
            n151 = Delete From Array(array=w444) -> (deleted portion=w439:string)  [unwired: 2 in, 1 out]
            n152 = call "Decode Publish Packet.vim"("Payload type"="", "PUBLISH"=w446, "Client in"=w445) -> ("Payload"=w434:string)  [unwired: 5 in, 3 out]
            n153 = Index Array(array=w437, index (col)=0 ("disabled index (col)")) -> (element=w440:string[])  [unwired: 1 in]
            n154 = Search 1D Array(1D array=w440, element=w439) -> (index of element=w438:i32)  [unwired: 1 in]
            n155 = Array Subset(array=w437, length (row)=50 ("length")) -> (w443:string[][])  [unwired: 3 in]
            n156 = case shown="Default" w438 {
              selector: w438 -> [_ w454]
              tunnel: [w451 w456] -> w436
              tunnel: w443 -> [w450 w457]
              tunnel: w434 -> [w449 w459]
              tunnel: w439 -> [w448 w458]
              frame -1 {
                n157 = Build Array(w448, w449, "" ("element")) -> (w452:string[])
                n158 = Build Array (concatenate)(w452, w450) -> (w451:string[][])
              }
              frame Default {
                n159 = Build Array(w458, w459, "" ("element")) -> (w455:string[])
                n160 = Replace Array Subset(array=w457, new element=w455, index (row)=w454) -> (w456:string[][])  [unwired: 1 in]
              }
            }
          }
          frame "disconnect" {
            n161 = Delete From Array(array=w470) -> (deleted portion=w465:string)  [unwired: 2 in, 1 out]
            n162 = call "Decode Publish Packet.vim"("Payload type"="", "PUBLISH"=w472, "Client in"=w471) -> ("Payload"=w460:string)  [unwired: 5 in, 3 out]
            n163 = Index Array(array=w463, index (col)=0 ("disabled index (col)")) -> (element=w466:string[])  [unwired: 1 in]
            n164 = Search 1D Array(1D array=w466, element=w465) -> (index of element=w464:i32)  [unwired: 1 in]
            n165 = Array Subset(array=w463, length (row)=50 ("length")) -> (w469:string[][])  [unwired: 3 in]
            n166 = case shown="Default" w464 {
              selector: w464 -> [_ w483]
              tunnel: [w477 w485] -> w462
              tunnel: w469 -> [w476 w484]
              tunnel: w460 -> [w473 w479]
              tunnel: w465 -> [w475 _]
              frame -1 {
                n167 = Build Array(w475, "" ("element"), w473) -> (w478:string[])
                n168 = Build Array (concatenate)(w478, w476) -> (w477:string[][])
              }
              frame Default {
                n169 = Index Array(array=w484, index (row)=w483) -> (element=w482:string[])  [unwired: 1 in]
                n170 = Replace Array Subset(array=w482, new element=w479, index=2) -> (w480:string[])
                n171 = Replace Array Subset(array=w484, new element=w480, index (row)=w483) -> (w485:string[][])  [unwired: 1 in]
              }
            }
          }
          frame "will" {
            n172 = Delete From Array(array=w497) -> (deleted portion=w492:string)  [unwired: 2 in, 1 out]
            n173 = call <vilib>:"Read Payload.vi"("ControlPacket in"=w487) -> ("Payload"=w488:u8[])  [unwired: 9 in, 1 out]
            n174 = Index Array(array=w490, index (col)=0 ("disabled index (col)")) -> (element=w493:string[])  [unwired: 1 in]
            n175 = Byte Array To String(unsigned byte array=w488) -> (string=w486:string)
            "Will Message" <- w486
            n176 = Search 1D Array(1D array=w493, element=w492) -> (index of element=w491:i32)  [unwired: 1 in]
            n177 = Array Subset(array=w490, length (row)=50 ("length")) -> (w496:string[][])  [unwired: 3 in]
            n178 = case shown="-1" w491 {
              selector: w491 -> [_ w506]
              tunnel: [w502 w508] -> w489
              tunnel: w496 -> [w501 w509]
              tunnel: w486 -> [w498 w504]
              tunnel: w492 -> [w500 w510]
              frame -1 {
                n179 = Build Array(w500, "" ("element"), w498) -> (w503:string[])
                n180 = Build Array (concatenate)(w503, w501) -> (w502:string[][])
              }
              frame Default {
                n181 = Build Array(w510, "" ("element"), w504) -> (w507:string[])
                n182 = Replace Array Subset(array=w509, new element=w507, index (row)=w506) -> (w508:string[][])  [unwired: 1 in]
              }
            }
          }
        }
        n183 = property on="State History" class="MCListbox (strict)"("ItemNames"=w411) -> ()  [unwired: 2 in, 2 out]
        n184 = call <vilib>:"Add State(s) to Queue__JKI_lib_State_Machine.vi"("State(s) in (\"\")"=w424) -> ("States Out"=w423:string)  [unwired: 14 in]
      }
      frame "MQTT: Disconnect" {
        n185 = Unbundle By Name(w518) -> ("Client"=w516:refnum<class "Client.lvclass">)
        n186 = call <vilib>:"Disconnect from Server.vi"("error in (no error)"=w511, "Client in"=w516) -> ("error out"=w512:errorcluster, "Client out"=w515:refnum<class "Client.lvclass">)  [unwired: 7 in, 1 out]
        n187 = call <vilib>:"Stop.vi"("error in (no error)"=w512, "MQTT_Base in"=w515) -> ("error out"=w513:errorcluster, "MQTT_Base out"=w514:refnum<class "Client.lvclass">)  [unwired: 7 in, 1 out]
        n188 = Bundle By Name(cluster=w518, "Client"=w514) -> (w519:T3)
        n189 = call <vilib>:"Add State(s) to Queue__JKI_lib_State_Machine.vi"("State(s) in (\"\")"=w521) -> ("States Out"=w520:string)  [unwired: 14 in]
      }
      frame "MQTT: Unregister" {
        n190 = Unregister For Events(event registration refnum=w525, error in=w524) -> (error out=w523:errorcluster)
        n191 = call <vilib>:"Add State(s) to Queue__JKI_lib_State_Machine.vi"("State(s) in (\"\")"=w527) -> ("States Out"=w526:string)  [unwired: 14 in]
      }
      frame "MQTT: Destroy Client" {
        n192 = Unbundle By Name(w532) -> ("Client"=w531:refnum<class "Client.lvclass">)
        n193 = call-dynamic "Destroy.vi"("error in (no error)"=w530, "MQTT_Base in"=w531) -> ("error out"=w529:errorcluster)  [unwired: 8 in, 1 out]
        n194 = call <vilib>:"Add State(s) to Queue__JKI_lib_State_Machine.vi"("State(s) in (\"\")"=w534) -> ("States Out"=w533:string)  [unwired: 14 in]
      }
    }
  }
